vi "DoesPathInvolveTack.vi"(9 "Suggested regime modification":i32, 10 "Current Sailing Regime":T1, 11 "Desired Sailing Regime":T1) -> (3 "Path involves tack?":bool)   [LabVIEW 2013]
doc: "This VI checks the desired and current headings against the suggested modification, then returns a boolean stating whether or not the boat will tack across the wind.\n\nEric Schneider, March 2014"
uses:
  Data/TypeDefs/Sailing Regimes.ctl
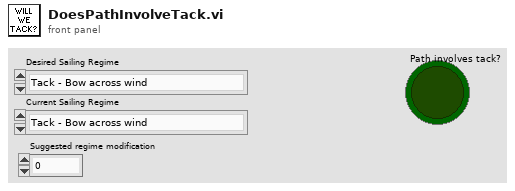
[diagram p1: front panel]
types:
  T1 = typedef "Sailing Regimes.ctl" = enum16{"Tack - Bow across wind", "Upwind - Starboard Tack", "Turn between Upwind/Reach - Starboard Tack", "Reach - Starboard Tack", "Turn between Reach/Run - Starboard Tack", "Run - Starboard Tack", "Jibe - Stern across wind", "Run - Port Tack", "Turn between Reach/Run - Port Tack", "Reach - Port Tack", "Turn between Upwind/Reach - Port Tack", "Upwind - Port Tack"}
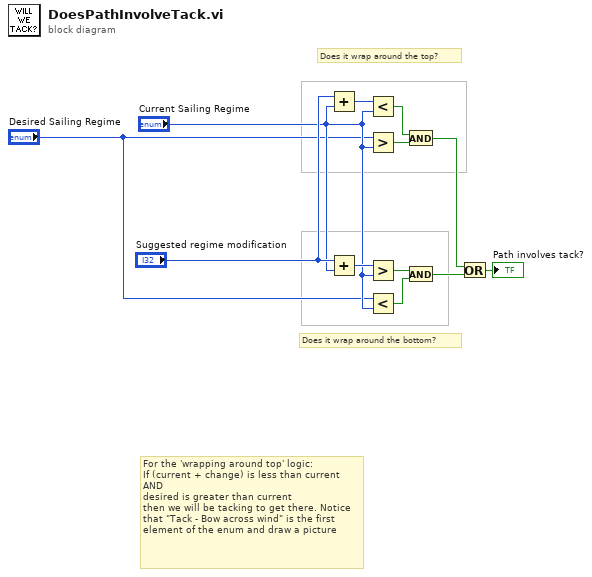
[diagram p0: block diagram]
diagram:
  # "Does it wrap around the bottom?"
  # "Does it wrap around the top?"
  # "For the 'wrapping around top' logic:\nIf (current + change) is less than current\nAND\ndesired is greater than current\nthen we will be tacking to get there. Notice that \"Tack - Bow across wind\" is the first element of the enum and draw a picture"
  n1 = Add(x="Suggested regime modification", y="Current Sailing Regime") -> (x+y=w12:i32)
  n2 = Add(x="Suggested regime modification", y="Current Sailing Regime") -> (x+y=w5:i32)
  n3 = Less?(x=w12, y="Current Sailing Regime") -> (x < y?=w11:bool)
  n4 = Greater?(x="Desired Sailing Regime", y="Current Sailing Regime") -> (0:w10:bool)
  n5 = Greater?(x=w5, y="Current Sailing Regime") -> (0:w6:bool)
  n6 = Less?(x="Desired Sailing Regime", y="Current Sailing Regime") -> (x < y?=w7:bool)
  n7 = And(x=w11, y=w10) -> (x .and. y?=w9:bool)
  n8 = And(x=w6, y=w7) -> (x .and. y?=w1:bool)
  n9 = Or(x=w9, y=w1) -> (x .or. y?=→"Path involves tack?":bool)
